vi "sub_balance.vi"(8 "error in":errorcluster) -> (0 "error out":errorcluster, 3 "Balance_xy":cluster{dbl, dbl}[](array[cluster]))   [LabVIEW 2016]
uses:
  ctl/UI_cmd-ctl.ctl
  ctl/Data_buf_cmd.ctl
  <vilib>/Waveform/WDTOps.llb/WDT Append Waveforms DBL.vi
  Global.vi
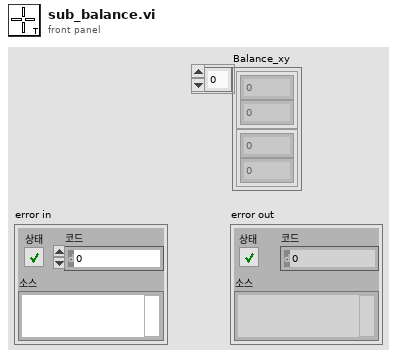
[diagram p1: front panel]
types:
  T1 = typedef "UI_cmd-ctl.ctl" = enum16{"default", "create", "read"}
  T2 = typedef "UI_ctl.ctl" = cluster{"Heater temp":refnum<vi>, "Heater chart":refnum<vi>, "vacuum (kpa)":refnum<vi>, "Balance xy graph":refnum<vi>, "Strain chart w cal":refnum<vi>, "Pickup force":refnum<vi>, "Pickup time":refnum<vi>, "Force chart":refnum<vi>, "Force graph T":refnum<vi>, "vacuum chart":refnum<vi>, "vacuum rt":refnum<vi>, "Strain raw graph":refnum<vi>, "Strain raw chart":refnum<vi>, "Bonding time":refnum<vi>, "Bonding force":refnum<vi>, "Balance":refnum<vi>, "Filtered force graph":refnum<vi>, "ROI intensity":refnum<vi>, "Heater_rt":refnum<vi>, "Detach force":refnum<vi>, "Force rt":refnum<vi>, "Mixed signal":refnum<vi>}
  T3 = typedef "Data_buf_cmd.ctl" = enum16{"insert", "default", "create", "clear"}
  T4 = typedef "data.ctl" = cluster{"Bonding force":dbl, "Bonding time":dbl, "Bonding index":dbl, "Pickup force":dbl, "Pickup time":dbl, "Pickup index":dbl, "Detach force":dbl, "Detach time":dbl, "Detach index":dbl, "Heater temp rt":dbl, "Vacuum rt":dbl, "IR raw data":i16[][], "IR temp data":dbl[][], "vacuum raw wf":waveform(dbl), "vacuum kpa wf":waveform(dbl), "strain raw wf":waveform(dbl)[], "Force rt":dbl, "Vacuum T":dbl, "Heater temp T":dbl, "Balance xy arrays":cluster{dbl, dbl}[], "Balance xy":cluster{dbl, dbl}[], "Bonding wf index":dbl, "Pickup wf index":dbl, "Bonding rising index":dbl, "Bonding falling index":dbl, "Pickup rising index":dbl, "Pickup falling index":dbl}
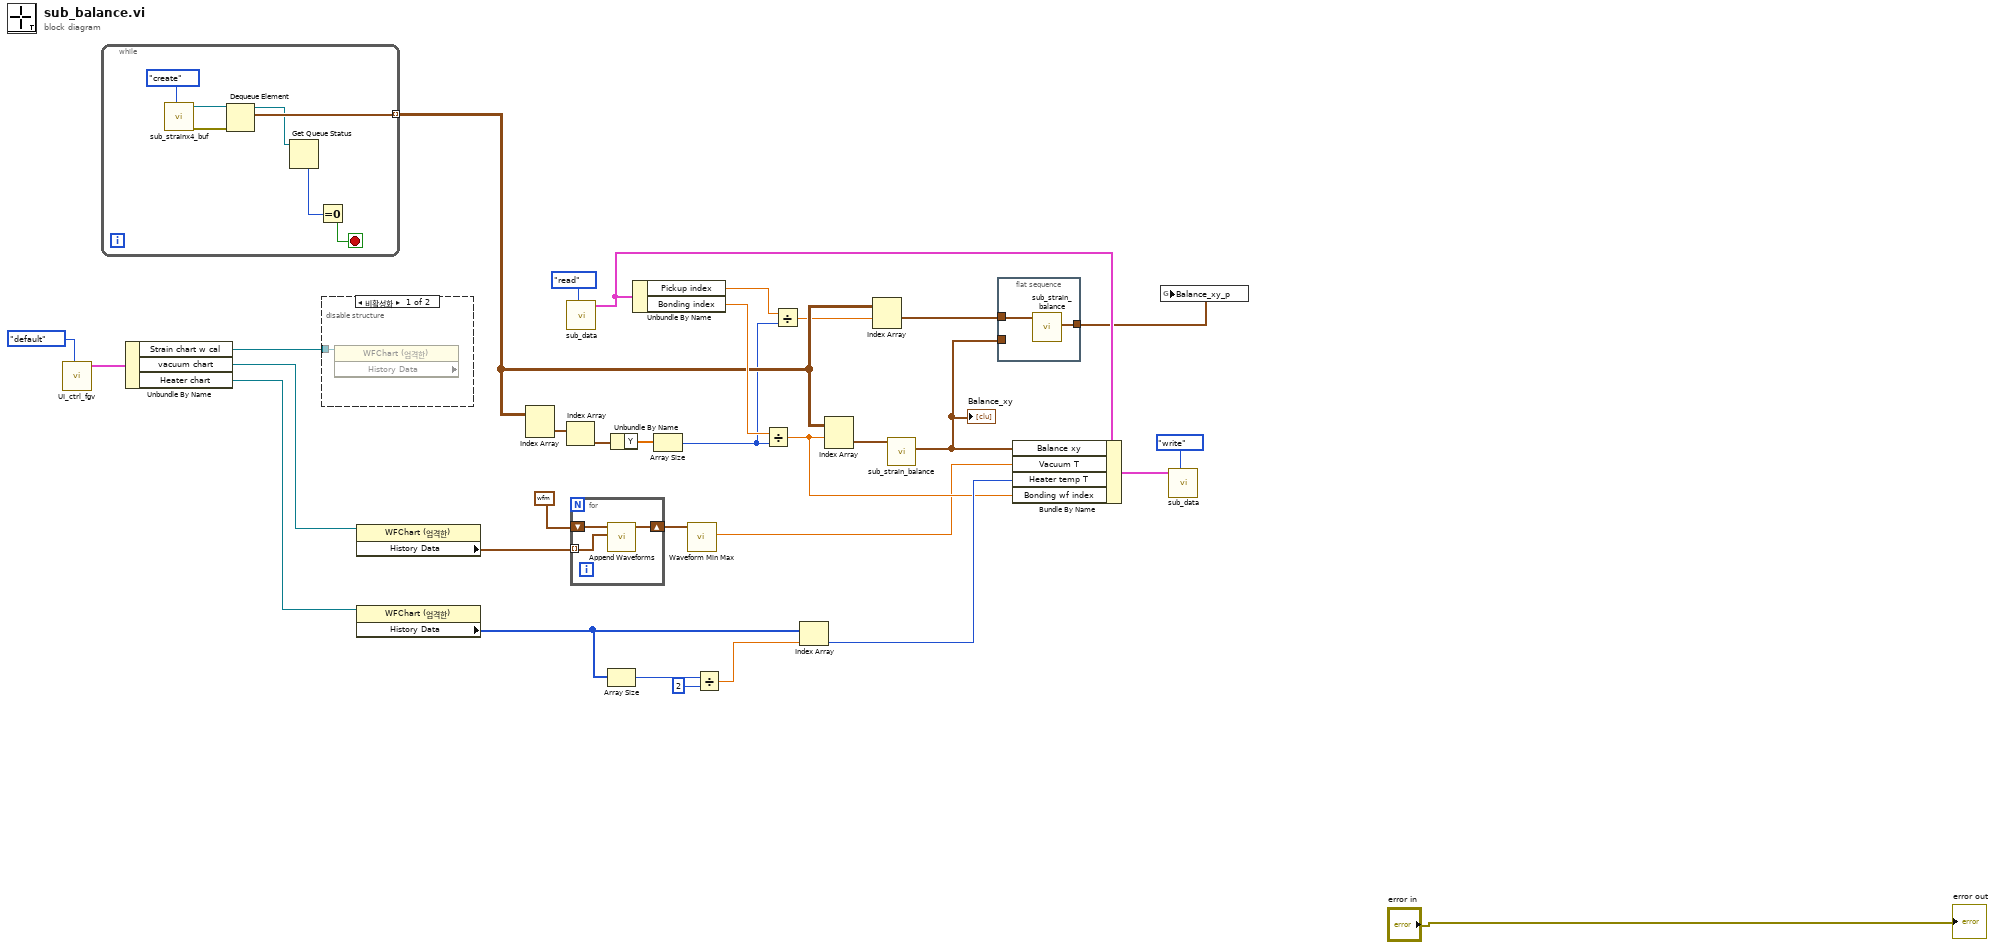
[diagram p0: block diagram]
diagram:
  n1 = call "UI_ctrl_fgv.vi"("cmd"=UI_cmd-ctl."default") -> ("UI cluster out"=w31:T2)  [unwired: 10 in]
  n2 = while {
    tunnel: [w39] -> w5 mode=indexing
    stop <- w37 stop-if-true
    n3 = call "sub_strainx4_buf.vi"("cmd"=Data_buf_cmd."create") -> ("error out"=w33:errorcluster, "queue out"=w34:refnum<queue>)  [unwired: 9 in]
    n4 = Dequeue Element(queue=w34, error in (no error)=w33) -> (queue out=w38:refnum<queue>, element=w39:waveform(dbl)[])  [unwired: 1 in, 2 out]
    n5 = Get Queue Status(queue=w38) -> (# elements in queue=w36:i32)  [unwired: 2 in, 7 out]
    n6 = Equal To 0?(x=w36) -> (x = 0?=w37:bool)
  }
  n7 = Unbundle By Name(w31) -> ("Strain chart w cal"=w30:refnum<vi>, "vacuum chart"=w25:refnum<vi>, "Heater chart"=w23:refnum<vi>)
  n8 = disable-structure shown="비활성화" {
    disable-tunnel: w30 -> [w40 _]
    frame Disabled {
      n9 = property class="WFChart (엄격한)" props=["History Data"](reference=w40) -> ()  [unwired: 1 in, 3 out]
    }
    frame Enabled {
    }
  }
  n10 = property class="WFChart (엄격한)"(reference=w25) -> ("History Data"=w15:waveform(dbl)[])  [unwired: 1 in, 2 out]
  n11 = property class="WFChart (엄격한)"(reference=w23) -> ("History Data"=w11:i32[])  [unwired: 1 in, 2 out]
  n12 = Index Array(array=w5) -> (element=w28:waveform(dbl)[])  [unwired: 2 in]
  n13 = Index Array(array=w28) -> (element=w27:waveform(dbl))  [unwired: 1 in]
  n14 = call "sub_data.vi"("cmd"=enum16{"ini", "write", "read"}."read") -> ("data out"=w19:T4)  [unwired: 9 in, 1 out]
  n15 = for {
    shift-right: [w41] -> w14
    shift-left: waveform(dbl) {"t0"=timestamp(0 s since 1904-01-01), "dt"=0.00024, "Y"=[]} -> [w43]
    tunnel: w15 -> [w42] mode=indexing
    n16 = call-poly <vilib>:"Append Waveforms.vi"("waveform B"=w42, "waveform A"=w43) -> ("waveform out"=w41:waveform(dbl))  [unwired: 8 in, 1 out]
  }
  n17 = Array Size(array=w11) -> (size(s)=w10:i32)
  n18 = Unbundle By Name(w27) -> ("Y"=w26:dbl[])
  n19 = Unbundle By Name(w19) -> ("Pickup index"=w3:dbl, "Bonding index"=w12:dbl)
  n20 = Array Size(array=w26) -> (size(s)=w2:i32)
  n21 = call <vilib>:"Waveform Min Max.vi"("waveform in"=w14) -> ("Y max"=w13:dbl)  [unwired: 5 in, 5 out]
  n22 = Divide(x=w10, y=2) -> (x/y=w8:dbl)
  n23 = Divide(x=w12, y=w2) -> (x/y=w17:dbl)
  n24 = Divide(x=w3, y=w2) -> (x/y=w1:dbl)
  n25 = Index Array(array=w11, index=w8) -> (element=w18:i32)
  n26 = Index Array(array=w5, index (row)=w17) -> (element=w20:waveform(dbl)[])  [unwired: 1 in]
  n27 = Index Array(array=w5, index (row)=w1) -> (element=w6:waveform(dbl)[])  [unwired: 1 in]
  n28 = call "sub_strain_balance.vi"("strain_offset_wf"=w20) -> ("Balance"=w7:cluster{"X":dbl, "Y":dbl}[])  [unwired: 9 in, 1 out]
  "Balance_xy" <- w7
  n29 = flat-sequence {
    tunnel: w7 -> [_]
    tunnel: w6 -> [w45]
    tunnel: [w44] -> w4
    frame #0 {
      n30 = call "sub_strain_balance.vi"("strain_offset_wf"=w45) -> ("Balance"=w44:cluster{"X":dbl, "Y":dbl}[])  [unwired: 9 in, 1 out]
    }
  }
  n31 = Bundle By Name(cluster=w19, "Balance xy"=w7, "Vacuum T"=w13, "Heater temp T"=w18, "Bonding wf index"=w17) -> (w21:T4)
  n32 = global write "Global.vi" "Balance_xy_p"(w4) -> ()
  n33 = call "sub_data.vi"("cmd"=enum16{"ini", "write", "read"}."write", "data in"=w21) -> ()  [unwired: 8 in, 2 out]
  "error out" <- "error in"
